vi "MU Load Register Ex.vi"(8 "error in (no error)":errorcluster, 9 "registerCount":u32=256, 10 "filepath":string, 11 "handle":u64) -> (0 "error out (no error)":errorcluster, 1 "valid":bool[](array[boolean]), 2 "values":u32[](array[numeric]), 3 "function return":u32)   [LabVIEW 2017, in "MU_3SL_interface.lvlib"]
uses:
  MU_3SL_interface.lvlib
  lib/MU_3SL_interface.dll
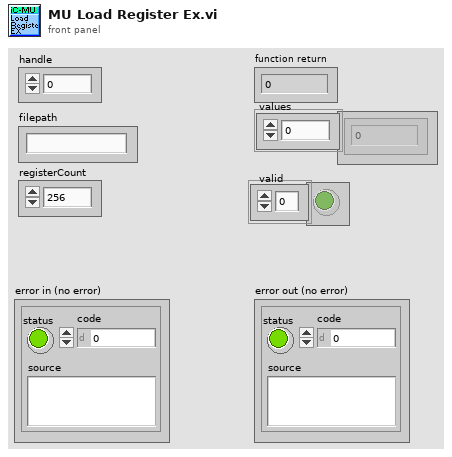
[diagram p1: front panel]
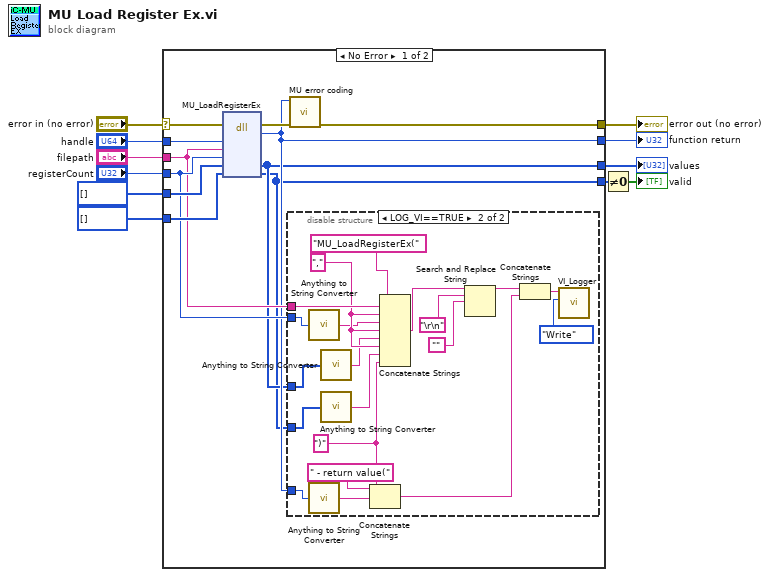
[diagram p0: block diagram]
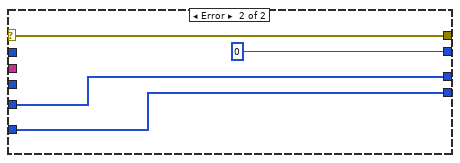
[diagram p3: hidden frame]
diagram:
  n1 = case shown="No Error" "error in (no error)" {
    selector: "error in (no error)" -> [w19 w46]
    tunnel: [w14 u32 0 ("return type")] -> w11
    tunnel: "handle" -> [w22 _]
    tunnel: [w20 w46] -> w9
    tunnel: "filepath" -> [w15 _]
    tunnel: "registerCount" -> [w16 _]
    tunnel: [w13 w44] -> w5
    tunnel: u32[] [] ("pulValid") -> [w18 w44]
    tunnel: u8[] [] ("valid") -> [w17 w43]
    tunnel: [w12 w43] -> w2
    frame No Error {
      n2 = dll-call lib="C:/Users/bes/AppData/Roaming/work/mu_9so/icsubmodules/soft_mu_3sl_master/lv_interface/lib/MU_3SL_interface**.*" fn="MU_LoadRegisterEx"(error in=w19, "handle"=w22, "filepath"=w15, "registerCount"=w16, "values"=w18, "valid"=w17) -> (error out=w21:errorcluster, "return type"=w14:u32, "values"=w13:u32[], "valid"=w12:u8[])  [unwired: 5 in, 1 out]
      n3 = disable-structure shown="LOG_VI==TRUE" {
        disable-tunnel: w14 -> [_ w24]
        disable-tunnel: w16 -> [_ w26]
        disable-tunnel: w15 -> [_ w37]
        disable-tunnel: w13 -> [_ w30]
        disable-tunnel: w12 -> [_ w28]
        frame condition #0 {
        }
        frame condition #1 (active) {
          w36 = ")" ("string")
          w31 = "," ("string")
          n4 = call "Anything to String Converter.vi"("anything"=w26) -> ("String"=w25:string)
          n5 = call "Anything to String Converter.vi"("anything"=w24) -> ("String"=w23:string)
          n6 = call "Anything to String Converter.vi"("anything"=w30) -> ("String"=w29:string)
          n7 = call "Anything to String Converter.vi"("anything"=w28) -> ("String"=w27:string)
          n8 = Concatenate Strings(" - return value(" ("string"), w23, w36) -> (w40:string)
          n9 = Concatenate Strings("MU_LoadRegisterEx(" ("Info in"), w37, w31, w25, w31, w29, w31, w27, w36) -> (w33:string)
          n10 = Search and Replace String(input string=w33, search string="\r\n", replace string="") -> (result string=w32:string)  [unwired: 5 in, 3 out]
          n11 = Concatenate Strings(w32, w40) -> (w39:string)
          n12 = call "VI_Logger.vi"("Action (Read)"=enum16{"Write", "Read"}."Write", "Info in"=w39) -> ()  [unwired: 8 in, 2 out]
        }
      }
      n13 = call "MU error coding.vi"("error in (no error)"=w21, "function return in"=w14) -> ("error out"=w20:errorcluster)  [unwired: 9 in]
    }
    frame Error {
    }
  }
  "function return" <- w11
  "error out (no error)" <- w9
  "values" <- w5
  n14 = Not Equal To 0?(x=w2) -> (x != 0?=→"valid":bool[])
